vi "Perform Action.vi"(7 "IPerform Action":refnum<class "Instrument.lvclass">, 8 "error in":errorcluster, 10 "Input":variant, 11 "Perform Action HSU MCU Read Strategy in":refnum<class "Perform Action HSU MCU Strategy.lvclass">) -> (0 "error out":errorcluster, 2 "Output":variant, 3 "Perform Action HSU MCU Read Strategy out":refnum<class "Perform Action HSU MCU Strategy.lvclass">)   [LabVIEW 2024, in "Perform Action HSU MCU Strategy.lvclass"]
uses:
  Perform Action HSU MCU Strategy.lvclass
  Instrument/Instrument.lvclass
  Perform Action HSU MCU Strategy.lvclass/Perform Action HSU MCU Strategy.ctl
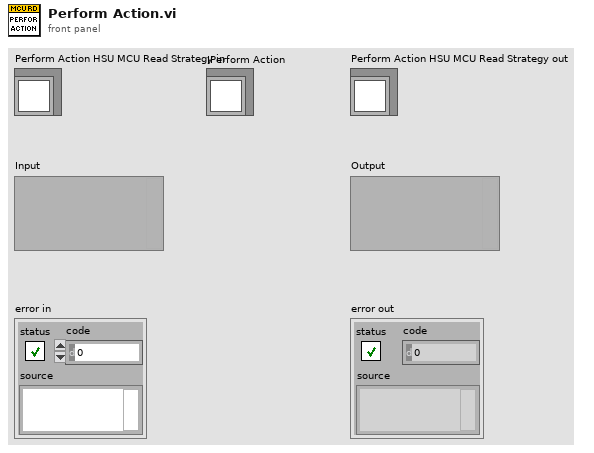
[diagram p1: front panel]
types:
  T1 = cluster{"Action":enum16{"Read", "Write"}, "MCU":string, "Attribute":string, "Value":variant}
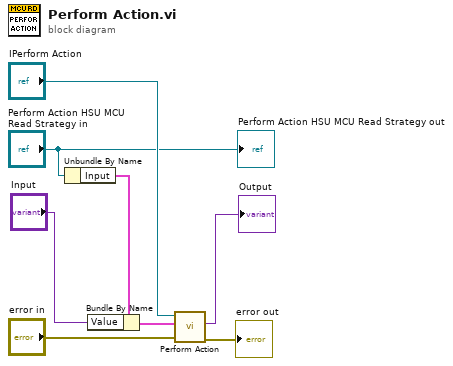
[diagram p0: block diagram]
diagram:
  n1 = Unbundle By Name("Perform Action HSU MCU Read Strategy in") -> ("Input"=w4:T1)
  n2 = Bundle By Name(cluster=w4, "Value"="Input") -> (w2:T1)
  n3 = call "Perform Action.vi"("Error In"="error in", "Input"=w2, "reference in"="IPerform Action") -> ("Error Out"=→"error out":errorcluster, "Output"=→"Output":variant)  [unwired: 6 in, 1 out]
  "Perform Action HSU MCU Read Strategy out" <- "Perform Action HSU MCU Read Strategy in"
